vi "练习1-控制信号发射器开关.vi"   [LabVIEW 2021]
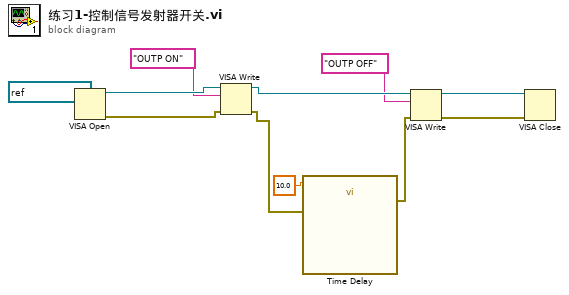
[diagram p0: block diagram]
diagram:
  n1 = VISA Open(VISA resource name=refnum<visa-resource-name> "DG1022U") -> (VISA resource name=w10:refnum<visa-resource-name>, error out=w9:errorcluster)  [unwired: 4 in]
  n2 = VISA Write(VISA resource name=w10, write buffer="OUTP ON", error in (no error)=w9) -> (VISA resource name out=w5:refnum<visa-resource-name>, error out=w7:errorcluster)  [unwired: 1 out]
  n3 = call "Time Delay"("error in (no error)"=w7, "Delay Time (s)"=10.0) -> ("error out"=w3:errorcluster)  [unwired: 9 in]
  n4 = VISA Write(VISA resource name=w5, write buffer="OUTP OFF", error in (no error)=w3) -> (VISA resource name out=w1:refnum<visa-resource-name>, error out=w2:errorcluster)  [unwired: 1 out]
  n5 = VISA Close(VISA resource name=w1, error in (no error)=w2) -> ()  [unwired: 1 out]
